vi "Threshold_v00.vi"(6 "MaxMin":T3, 8 "Lock Monitor":T2, 11 "Signals":T12={"Cavity Errors"={"OPO A"=0, "OPO B"=0, "MCC"=0, "Doubler"=0}, "Cavity Monitors"={"OPO A Monitor"=0, "OPO B Monitor"=0, "MCC Monitor"=0, "Doubler Monitor"=0}, "Lock Thresh"={"OPO A"=0, "OPO B"=0, "MCC"=0, "Doubler"=0}, "Re-Scan Thresh"={"OPO A"=0, "OPO B"=0, "MCC"=0, "Doubler"=0}, "PII In 1"={"Lock"=FALSE, "Hold"=FALSE, "P Gain"=0, "P BS"=-5, "I Gain"=0, "I BS"=-10, "I2 G"=0, "I2 BS"=-26, "Scan Amp"=0, "Scan Off"=0, "Scan FS"=0, "SFS BS"=0, "I Max value"=10000, "I2 Max value"=10000, "Scope.Offset"=0, "Trigger Direction"=enum."either", "Scan-PII thresh"=0}, "PII In 2"={"Lock"=FALSE, "Hold"=FALSE, "P Gain"=0, "P BS"=-10, "I Gain"=0, "I BS"=-10, "I2 G"=0, "I2 BS"=-26, "Scan Amp"=0, "Scan Off"=0, "Scan FS"=0, "SFS BS"=0, "I Max value"=10000, "I2 Max value"=10000, "Scope.Offset"=0, "Trigger Direction"=enum."either", "Scan-PII thresh"=0}, "PII In 3"={"Lock"=FALSE, "Hold"=FALSE, "P Gain"=0, "P BS"=-10, "I Gain"=0, "I BS"=-10, "I2 G"=0, "I2 BS"=-26, "Scan Amp"=0, "Scan Off"=0, "Scan FS"=0, "SFS BS"=0, "I Max value"=10000, "I2 Max value"=10000, "Scope.Offset"=0, "Trigger Direction"=enum."either", "Scan-PII thresh"=0}, "PII In 4"={"Lock"=FALSE, "Hold"=FALSE, "P Gain"=0, "P BS"=-10, "I Gain"=0, "I BS"=-10, "I2 G"=0, "I2 BS"=-26, "Scan Amp"=0, "Scan Off"=0, "Scan FS"=0, "SFS BS"=0, "I Max value"=10000, "I2 Max value"=10000, "Scope.Offset"=0, "Trigger Direction"=enum."either", "Scan-PII thresh"=0}, "Safety First"={"lim reset"=FALSE, "no limit"=FALSE, "pos slew rate * dt"=10, "neg slew rate * dt"=-10, "Hold All"=FALSE, "Count(Ticks)"=0}}) -> (3 "Control Cavity Cluster":T7={"Control A"={"Lock"=FALSE, "Hold"=FALSE, "P Gain"=0, "P BS"=-5, "I Gain"=0, "I BS"=-10, "I2 G"=0, "I2 BS"=-26, "Scan Amp"=0, "Scan Off"=0, "Scan FS"=0, "SFS BS"=0, "I Max value"=10000, "I2 Max value"=10000, "Scope.Offset"=0, "Trigger Direction"=enum."either", "Scan-PII thresh"=0}, "Control B"={"Lock"=FALSE, "Hold"=FALSE, "P Gain"=0, "P BS"=-5, "I Gain"=0, "I BS"=-10, "I2 G"=0, "I2 BS"=-26, "Scan Amp"=0, "Scan Off"=0, "Scan FS"=0, "SFS BS"=0, "I Max value"=10000, "I2 Max value"=10000, "Scope.Offset"=0, "Trigger Direction"=enum."either", "Scan-PII thresh"=0}, "Control MCC"={"Lock"=FALSE, "Hold"=FALSE, "P Gain"=0, "P BS"=-5, "I Gain"=0, "I BS"=-10, "I2 G"=0, "I2 BS"=-26, "Scan Amp"=0, "Scan Off"=0, "Scan FS"=0, "SFS BS"=0, "I Max value"=10000, "I2 Max value"=10000, "Scope.Offset"=0, "Trigger Direction"=enum."either", "Scan-PII thresh"=0}, "Control Doubler"={"Lock"=FALSE, "Hold"=FALSE, "P Gain"=0, "P BS"=-5, "I Gain"=0, "I BS"=-10, "I2 G"=0, "I2 BS"=-26, "Scan Amp"=0, "Scan Off"=0, "Scan FS"=0, "SFS BS"=0, "I Max value"=10000, "I2 Max value"=10000, "Scope.Offset"=0, "Trigger Direction"=enum."either", "Scan-PII thresh"=0}, "Lock Point?"={"OPO A"=FALSE, "OPO B"=FALSE, "MCC"=FALSE, "Doubler"=FALSE}, "Re-scan?"={"OPO A"=FALSE, "OPO B"=FALSE, "MCC"=FALSE, "Doubler"=FALSE}, "Cavity Errors"={"OPO A"=0, "OPO B"=0, "MCC"=0, "Doubler"=0}, "Max"={"Max OPO A"=0, "Max OPO B"=0, "Max MCC"=0, "Max Doubler"=0}, "Min"={"Min OPO A"=0, "Min OPO B"=0, "Min MCC"=0, "Min Doubler"=0}, "Lock Threshold"={"Thresh OPO A "=0, "Thresh OPO B"=0, "Thresh MCC"=0, "Thresh Doubler"=0}, "Re-Scan Threshold"={"Thresh OPO A "=0, "Thresh OPO B"=0, "Thresh MCC"=0, "Thresh Doubler"=0}, "State (-1)"={"OPO A"=enum."Safe", "OPO B"=enum."Safe", "MCC"=enum."Safe", "Doubler"=enum."Safe"}, "Lock pressed? (-1)"={"OPO A"=FALSE, "OPO B"=FALSE, "MCC"=FALSE, "Doubler"=FALSE}, "Safety First"={"lim reset"=FALSE, "no limit"=FALSE, "pos slew rate * dt"=0, "neg slew rate * dt"=0, "Hold All"=FALSE, "Count(Ticks)"=0}}, 5 "Unlocked?(T=yes)":T1)   [LabVIEW 2010]
doc: "Determines if the cavity is on resonance by comparing the DC monitor to a user-defined threshold."
uses:
  Strict Type Defs/Signals.ctl
  Strict Type Defs/Cavity Errors.ctl
  Strict Type Defs/Cavity Monitors.ctl
  Strict Type Defs/Lock Thresh.ctl
  Strict Type Defs/PII individual.ctl
  Strict Type Defs/Safety First.ctl
  Strict Type Defs/Control Cavity Cluster.ctl
  Strict Type Defs/Lock Point.ctl
  Strict Type Defs/Re-Scan.ctl
  Strict Type Defs/Max.ctl
  Strict Type Defs/Min.ctl
  Strict Type Defs/MaxMin.ctl
panel:
  in  "Control Cavity Cluster":T7={"Control A"={"Lock"=FALSE, "Hold"=FALSE, "P Gain"=0, "P BS"=-5, "I Gain"=0, "I BS"=-10, "I2 G"=0, "I2 BS"=-26, "Scan Amp"=0, "Scan Off"=0, "Scan FS"=0, "SFS BS"=0, "I Max value"=10000, "I2 Max value"=10000, "Scope.Offset"=0, "Trigger Direction"=enum."either", "Scan-PII thresh"=0}, "Control B"={"Lock"=FALSE, "Hold"=FALSE, "P Gain"=0, "P BS"=-5, "I Gain"=0, "I BS"=-10, "I2 G"=0, "I2 BS"=-26, "Scan Amp"=0, "Scan Off"=0, "Scan FS"=0, "SFS BS"=0, "I Max value"=10000, "I2 Max value"=10000, "Scope.Offset"=0, "Trigger Direction"=enum."either", "Scan-PII thresh"=0}, "Control MCC"={"Lock"=FALSE, "Hold"=FALSE, "P Gain"=0, "P BS"=-5, "I Gain"=0, "I BS"=-10, "I2 G"=0, "I2 BS"=-26, "Scan Amp"=0, "Scan Off"=0, "Scan FS"=0, "SFS BS"=0, "I Max value"=10000, "I2 Max value"=10000, "Scope.Offset"=0, "Trigger Direction"=enum."either", "Scan-PII thresh"=0}, "Control Doubler"={"Lock"=FALSE, "Hold"=FALSE, "P Gain"=0, "P BS"=-5, "I Gain"=0, "I BS"=-10, "I2 G"=0, "I2 BS"=-26, "Scan Amp"=0, "Scan Off"=0, "Scan FS"=0, "SFS BS"=0, "I Max value"=10000, "I2 Max value"=10000, "Scope.Offset"=0, "Trigger Direction"=enum."either", "Scan-PII thresh"=0}, "Lock Point?"={"OPO A"=FALSE, "OPO B"=FALSE, "MCC"=FALSE, "Doubler"=FALSE}, "Re-scan?"={"OPO A"=FALSE, "OPO B"=FALSE, "MCC"=FALSE, "Doubler"=FALSE}, "Cavity Errors"={"OPO A"=0, "OPO B"=0, "MCC"=0, "Doubler"=0}, "Max"={"Max OPO A"=0, "Max OPO B"=0, "Max MCC"=0, "Max Doubler"=0}, "Min"={"Min OPO A"=0, "Min OPO B"=0, "Min MCC"=0, "Min Doubler"=0}, "Lock Threshold"={"Thresh OPO A "=0, "Thresh OPO B"=0, "Thresh MCC"=0, "Thresh Doubler"=0}, "Re-Scan Threshold"={"Thresh OPO A "=0, "Thresh OPO B"=0, "Thresh MCC"=0, "Thresh Doubler"=0}, "State (-1)"={"OPO A"=enum."Safe", "OPO B"=enum."Safe", "MCC"=enum."Safe", "Doubler"=enum."Safe"}, "Lock pressed? (-1)"={"OPO A"=FALSE, "OPO B"=FALSE, "MCC"=FALSE, "Doubler"=FALSE}, "Safety First"={"lim reset"=FALSE, "no limit"=FALSE, "pos slew rate * dt"=0, "neg slew rate * dt"=0, "Hold All"=FALSE, "Count(Ticks)"=0}}
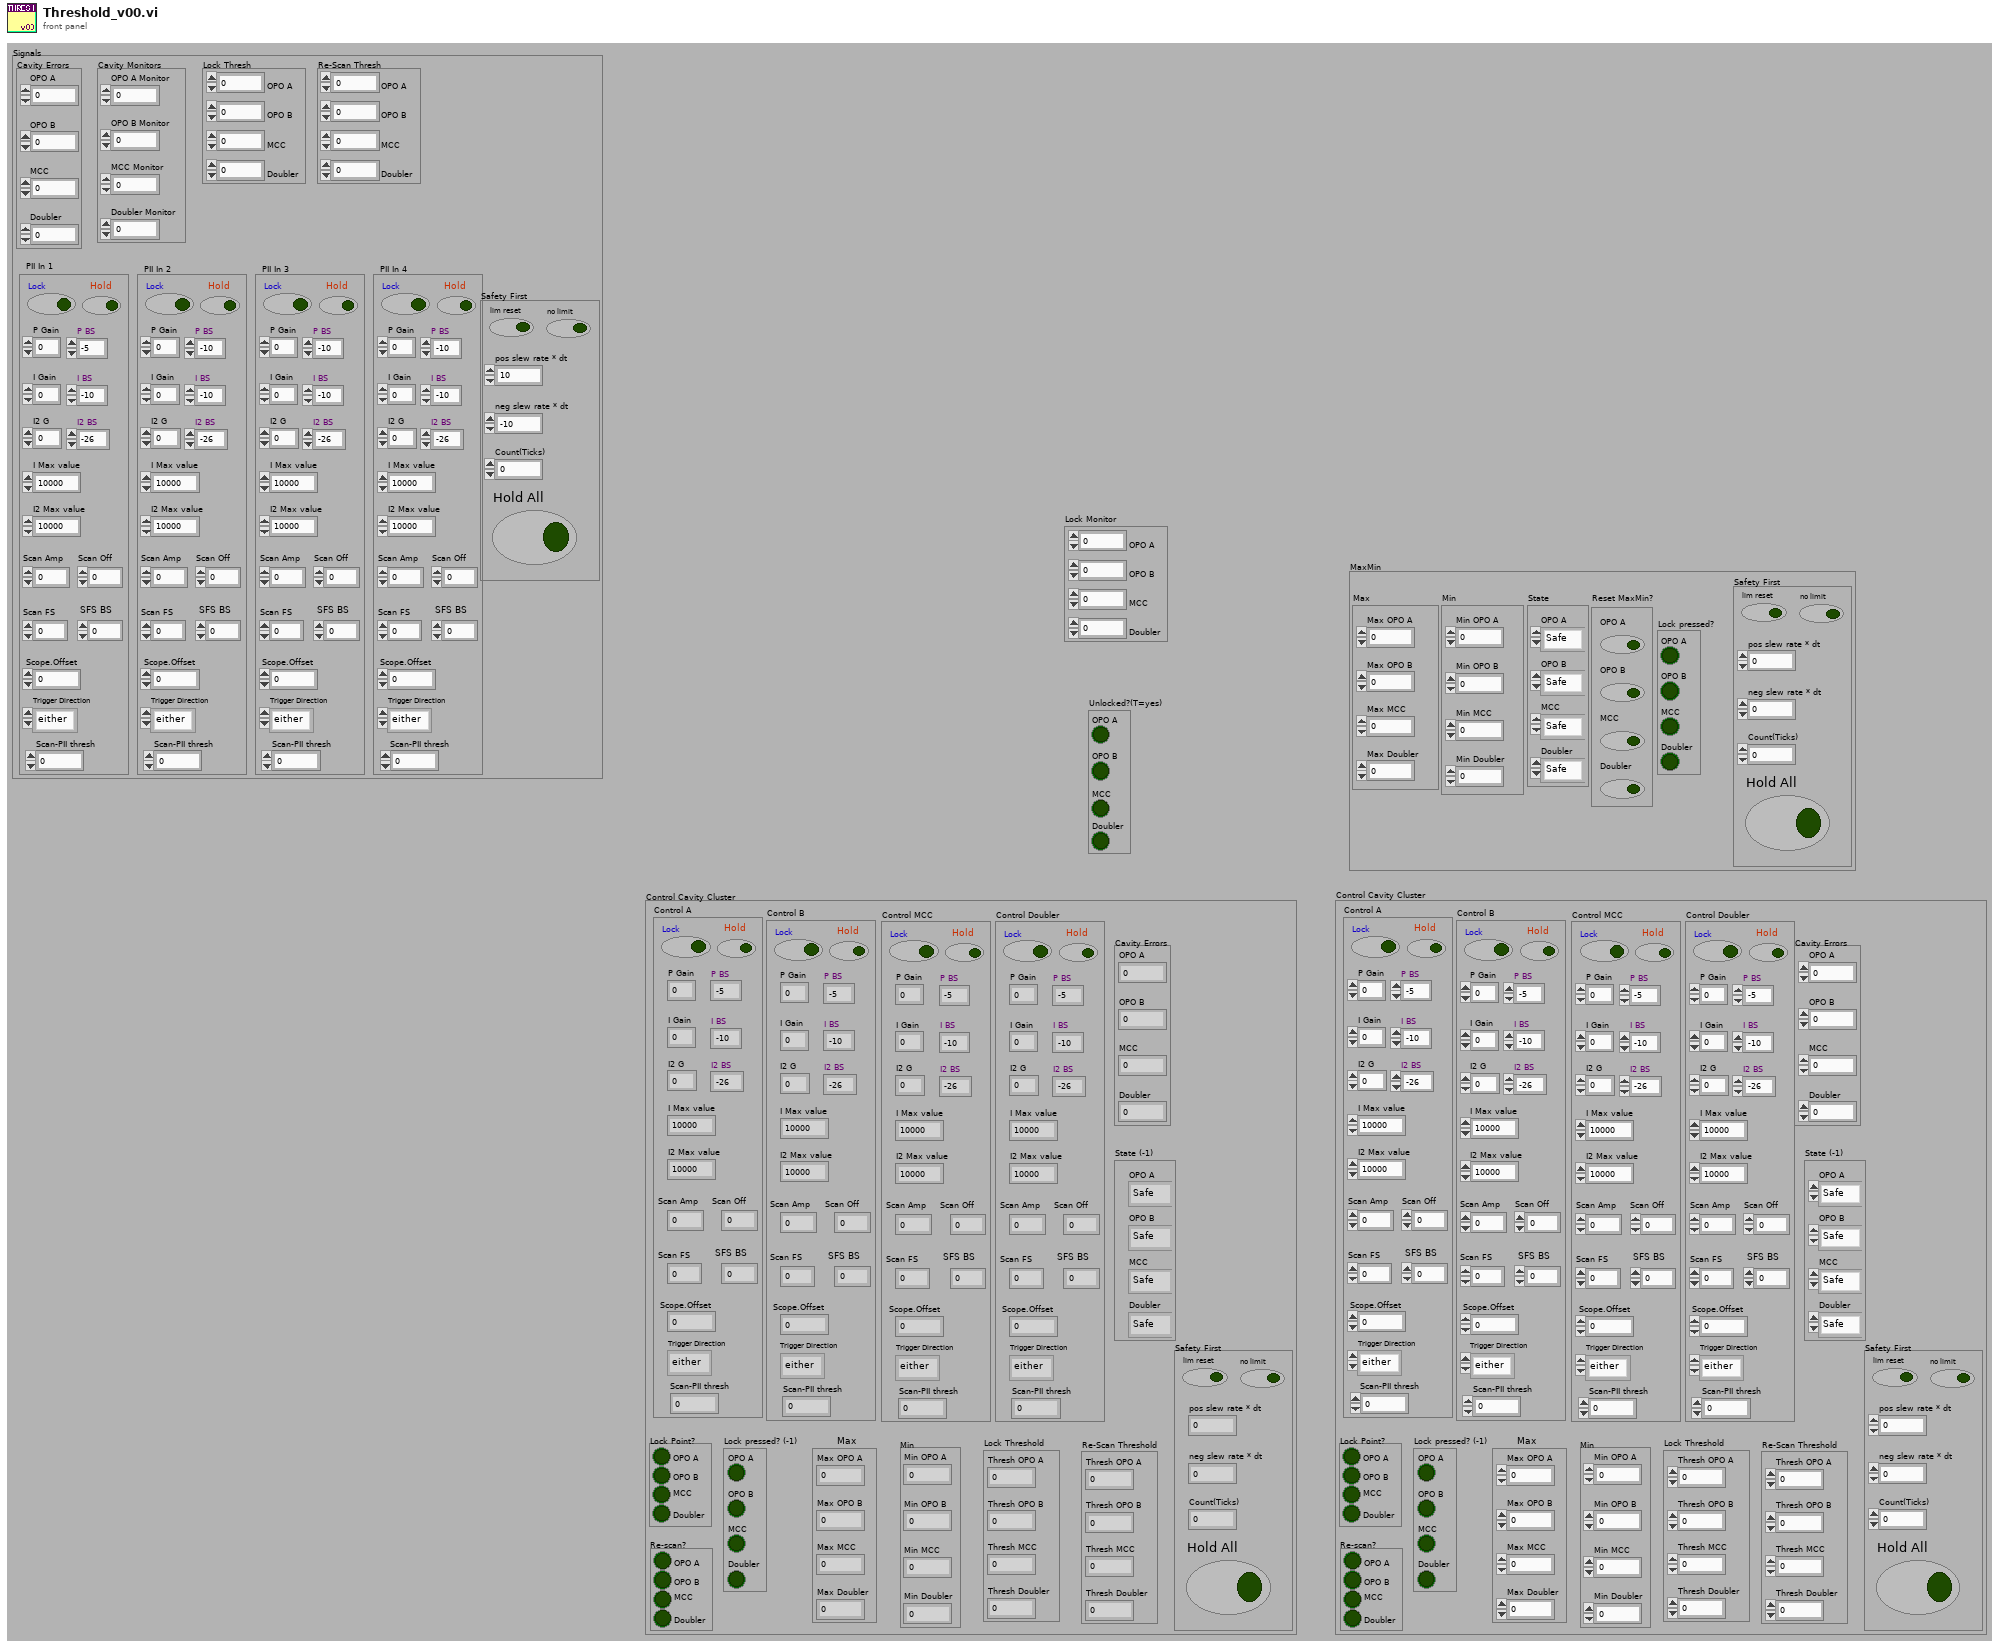
[diagram p1: front panel]
types:
  T1 = cluster{"OPO A":bool, "OPO B":bool, "MCC":bool, "Doubler":bool}
  T2 = cluster{"OPO A":i16, "OPO B":i16, "MCC":i16, "Doubler":i16}
  T3 = typedef "MaxMin.ctl" = cluster{"State":cluster{"OPO A":enum16{"Safe", "Hold", "Scan", "Lock"}, "OPO B":enum16{"Safe", "Hold", "Scan", "Lock"}, "MCC":enum16{"Safe", "Hold", "Scan", "Lock"}, "Doubler":enum16{"Safe", "Hold", "Scan", "Lock"}}, "Reset MaxMin?":cluster{"OPO A":bool, "OPO B":bool, "MCC":bool, "Doubler":bool}, "Max":T4, "Min":T5, "Lock pressed?":cluster{"OPO A":bool, "OPO B":bool, "MCC":bool, "Doubler":bool}, "Safety First":T6}
  T4 = typedef "Max.ctl" = cluster{"Max OPO A":i16, "Max OPO B":i16, "Max MCC":i16, "Max Doubler":i16}
  T5 = typedef "Min.ctl" = cluster{"Min OPO A":i16, "Min OPO B":i16, "Min MCC":i16, "Min Doubler":i16}
  T6 = typedef "Safety First.ctl" = cluster{"lim reset":bool, "no limit":bool, "pos slew rate * dt":i16, "neg slew rate * dt":i16, "Hold All":bool, "Count(Ticks)":u32}
  T7 = typedef "Control Cavity Cluster.ctl" = cluster{"Control A":T8, "Control B":T8, "Control MCC":T8, "Control Doubler":T8, "Lock Point?":T9, "Re-scan?":T10, "Cavity Errors":T11, "Max":T4, "Min":T5, "Lock Threshold":cluster{"Thresh OPO A ":i16, "Thresh OPO B":i16, "Thresh MCC":i16, "Thresh Doubler":i16}, "Re-Scan Threshold":cluster{"Thresh OPO A ":i16, "Thresh OPO B":i16, "Thresh MCC":i16, "Thresh Doubler":i16}, "State (-1)":cluster{"OPO A":enum16{"Safe", "Hold", "Scan", "Lock"}, "OPO B":enum16{"Safe", "Hold", "Scan", "Lock"}, "MCC":enum16{"Safe", "Hold", "Scan", "Lock"}, "Doubler":enum16{"Safe", "Hold", "Scan", "Lock"}}, "Lock pressed? (-1)":cluster{"OPO A":bool, "OPO B":bool, "MCC":bool, "Doubler":bool}, "Safety First":T6}
  T8 = typedef "PII individual.ctl" = cluster{"Lock":bool, "Hold":bool, "P Gain":i32, "P BS":i16, "I Gain":i32, "I BS":i16, "I2 G":i32, "I2 BS":i16, "Scan Amp":i16, "Scan Off":i16, "Scan FS":u16, "SFS BS":i16, "I Max value":i32, "I2 Max value":i32, "Scope.Offset":i16, "Trigger Direction":enum8{"either", "minus-plus", "plus-minus"}, "Scan-PII thresh":i16}
  T9 = typedef "Lock Point.ctl" = cluster{"OPO A":bool, "OPO B":bool, "MCC":bool, "Doubler":bool}
  T10 = typedef "Re-Scan.ctl" = cluster{"OPO A":bool, "OPO B":bool, "MCC":bool, "Doubler":bool}
  T11 = typedef "Cavity Errors.ctl" = cluster{"OPO A":i16, "OPO B":i16, "MCC":i16, "Doubler":i16}
  T12 = typedef "Signals.ctl" = cluster{"Cavity Errors":T11, "Cavity Monitors":T13, "Lock Thresh":T14, "Re-Scan Thresh":T14, "PII In 1":T8, "PII In 2":T8, "PII In 3":T8, "PII In 4":T8, "Safety First":T6}
  T13 = typedef "Cavity Monitors.ctl" = cluster{"OPO A Monitor":i16, "OPO B Monitor":i16, "MCC Monitor":i16, "Doubler Monitor":i16}
  T14 = typedef "Lock Thresh.ctl" = cluster{"OPO A":i16, "OPO B":i16, "MCC":i16, "Doubler":i16}
  T15 = cluster{"OPO A":enum16{"Safe", "Hold", "Scan", "Lock"}, "OPO B":enum16{"Safe", "Hold", "Scan", "Lock"}, "MCC":enum16{"Safe", "Hold", "Scan", "Lock"}, "Doubler":enum16{"Safe", "Hold", "Scan", "Lock"}}
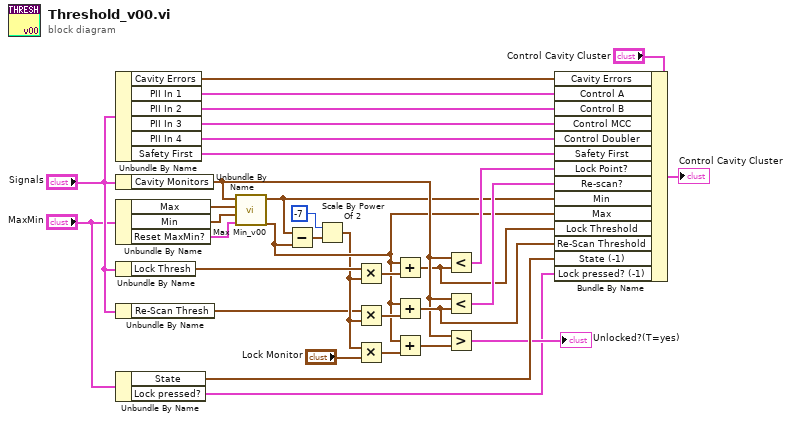
[diagram p0: block diagram]
diagram:
  n1 = Unbundle By Name("Signals") -> ("Cavity Errors"=w21:T11, "PII In 1"=w20:T8, "PII In 2"=w19:T8, "PII In 3"=w18:T8, "PII In 4"=w17:T8, "Safety First"=w25:T6)
  n2 = Unbundle By Name("Signals") -> ("Cavity Monitors"=w11:T13)
  n3 = Unbundle By Name("MaxMin") -> ("Max"=w33:T4, "Min"=w32:T5, "Reset MaxMin?"=w8:T1)
  n4 = Unbundle By Name("Signals") -> ("Lock Thresh"=w3:T14)
  n5 = Unbundle By Name("Signals") -> ("Re-Scan Thresh"=w1:T14)
  n6 = Unbundle By Name("MaxMin") -> ("State"=w15:T15, "Lock pressed?"=w4:T1)
  n7 = call "Max Min_v00.vi"("Reset MaxMin?"=w8, "Min (-1)"=w32, "Max (-1)"=w33, "Cavity Monitors"=w11) -> ("Max"=w6:T4, "Min"=w7:T5)  [unwired: 6 in]
  n8 = Subtract(x=w7, y=w6) -> (x-y=w30:T5)
  n9 = Scale By Power Of 2(n=-7, x=w30) -> (x*2^n=w2:T5)
  n10 = Multiply(x=w3, y=w2) -> (x*y=w29:T14)
  n11 = Multiply(x=w1, y=w2) -> (x*y=w28:T14)
  n12 = Multiply(x=w2, y="Lock Monitor") -> (x*y=w12:T5)
  n13 = Add(x=w6, y=w29) -> (x+y=w5:T4)
  n14 = Add(x=w6, y=w28) -> (x+y=w16:T4)
  n15 = Add(x=w6, y=w12) -> (x+y=w13:T4)
  n16 = Less?(x=w11, y=w5) -> (x < y?=w24:cluster{bool, bool, bool, bool})
  n17 = Less?(x=w11, y=w16) -> (x < y?=w23:cluster{bool, bool, bool, bool})
  n18 = Greater?(x=w11, y=w13) -> (0:→"Unlocked?(T=yes)":cluster{bool, bool, bool, bool})
  n19 = Bundle By Name(cluster="Control Cavity Cluster", "Cavity Errors"=w21, "Control A"=w20, "Control B"=w19, "Control MCC"=w18, "Control Doubler"=w17, "Safety First"=w25, "Lock Point?"=w24, "Re-scan?"=w23, "Min"=w7, "Max"=w6, "Lock Threshold"=w5, "Re-Scan Threshold"=w16, "State (-1)"=w15, "Lock pressed? (-1)"=w4) -> (→"Control Cavity Cluster":T7)
